vi "Create Library Folder.vi"(11 "Actor Script Strategy in":refnum<class "Actor Script Strategy.lvclass">) -> (3 "Actor Script Strategy out":refnum<class "Actor Script Strategy.lvclass">)   [LabVIEW 2021, in "_Create From Template.lvlib" / "Script Strategy.lvlib" / "Actor Script Strategy.lvclass"]
uses:
  Actor Script Strategy.lvclass
  Actor Script Strategy.lvclass/Actor Script Strategy.ctl
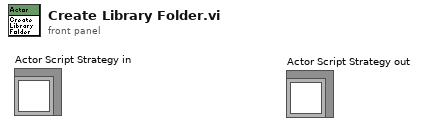
[diagram p1: front panel]
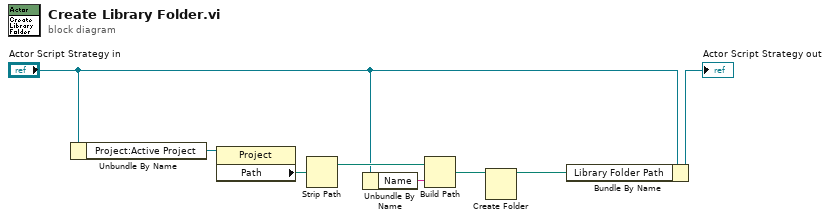
[diagram p0: block diagram]
diagram:
  n1 = Unbundle By Name("Actor Script Strategy in") -> ("Project:Active Project"=w3:refnum<vi>)
  n2 = property class="Project"(reference=w3) -> ("Path"=w6:path)  [unwired: 1 in, 2 out]
  n3 = Strip Path(path=w6) -> (stripped path=w7:path)  [unwired: 1 out]
  n4 = Unbundle By Name("Actor Script Strategy in") -> ("Name"=w5:string)
  n5 = Build Path(base path=w7, name or relative path=w5) -> (appended path=w8:path)
  n6 = Create Folder(path (use dialog)=w8) -> (created path=w1:path)  [unwired: 2 in, 2 out]
  n7 = Bundle By Name(cluster="Actor Script Strategy in", "Library Folder Path"=w1) -> (→"Actor Script Strategy out":refnum<class "Actor Script Strategy.lvclass">)
